vi "Render.vi"(8 "error in (no error)":errorcluster, 11 "XRay Axis Rails in":refnum<class "XRay Axis Rails.lvclass">) -> (0 "error out":errorcluster, 2 "Scene Object":refnum<vi>, 3 "XRay Axis Rails out":refnum<class "XRay Axis Rails.lvclass">)   [LabVIEW 2026, in "XRay Axis Rails.lvclass"]
uses:
  XRay Axis Rails.lvclass
  XRay Axis Rails.lvclass/XRay Axis Rails.ctl
  <vilib>/picture/picture.llb/imagedata.ctl
  <vilib>/picture/3D Picture Control/Object/Create Object (drawable).vi
  <vilib>/picture/3D Picture Control/Object/Add Object (reference).vi
  <vilib>/picture/3D Picture Control/Helpers/Apply Texture (reference).vi
  <vilib>/picture/3D Picture Control/NI_3D Picture Control.lvlib
panel:
  in  "Apply Mode":T1(ring)=enum."As a replacement"
  in  "error in (no error) 2":errorcluster
  in  "Translation 4":cluster{"X":sgl, "Y":sgl, "Z":sgl}={"X"=0.0, "Y"=9.0, "Z"=5.0}
  in  "Translation 3":cluster{"X":sgl, "Y":sgl, "Z":sgl}={"X"=0.0, "Y"=5.0, "Z"=5.0}
  in  "Translation 2":cluster{"X":sgl, "Y":sgl, "Z":sgl}={"X"=7.0, "Y"=7.5, "Z"=0.0}
  in  "Translation":cluster{"X":sgl, "Y":sgl, "Z":sgl}={"X"=4.0, "Y"=7.5, "Z"=0.0}
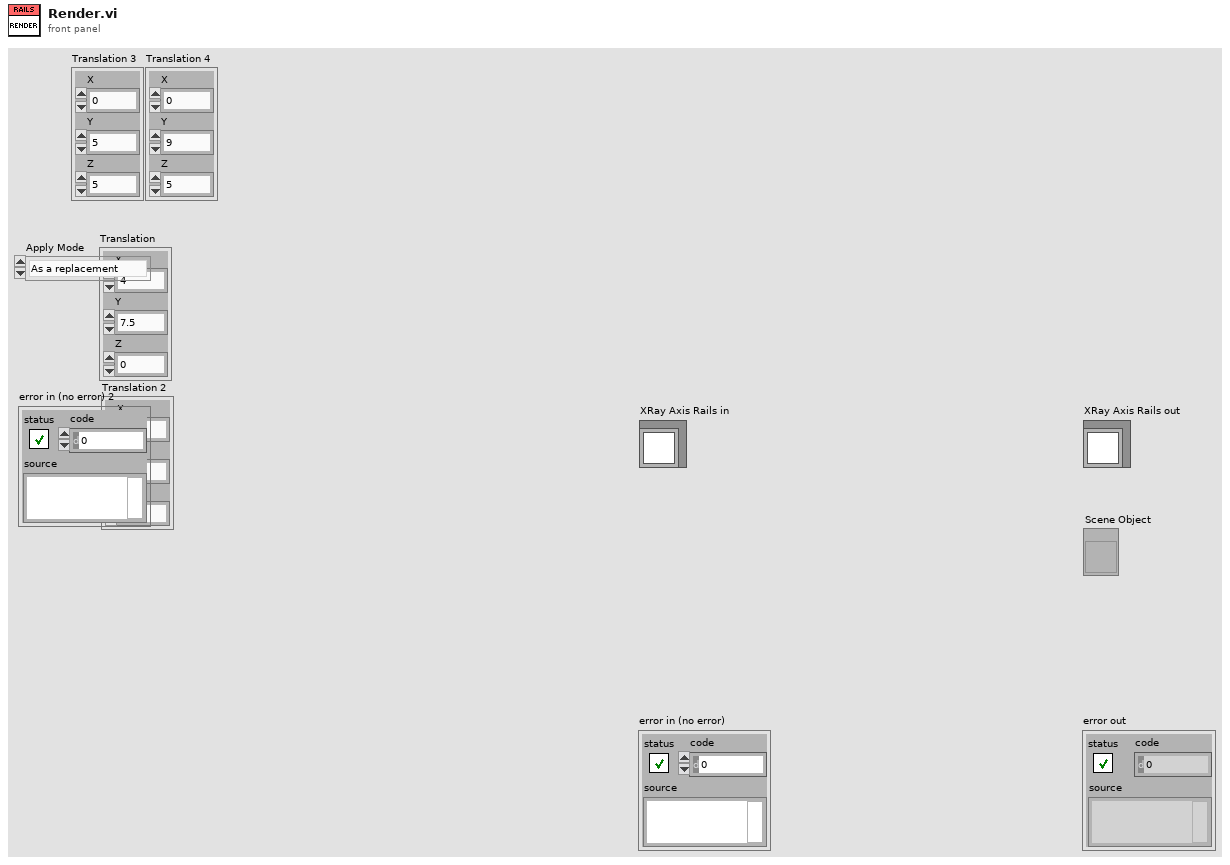
[diagram p1: front panel]
types:
  T1 = enum16{"As a Decal", "With Modulation", "With Blending", "As a replacement"}
  T2 = enum16{"No Filtration", "Linear Filtration", "Simple Mipmap Filtration", "Bilinear Filtration", "Trilinear Filtration"}
  T3 = enum16{"Inherit Value", "Points", "Wireframe", "Polygons"}
  T4 = typedef "imagedata.ctl" = cluster{"image type":i32, "image depth":i32, "image":u8[], "mask":u8[], "colors":u32[], "Rectangle":cluster{"left":i16, "top":i16, "right":i16, "bottom":i16}}
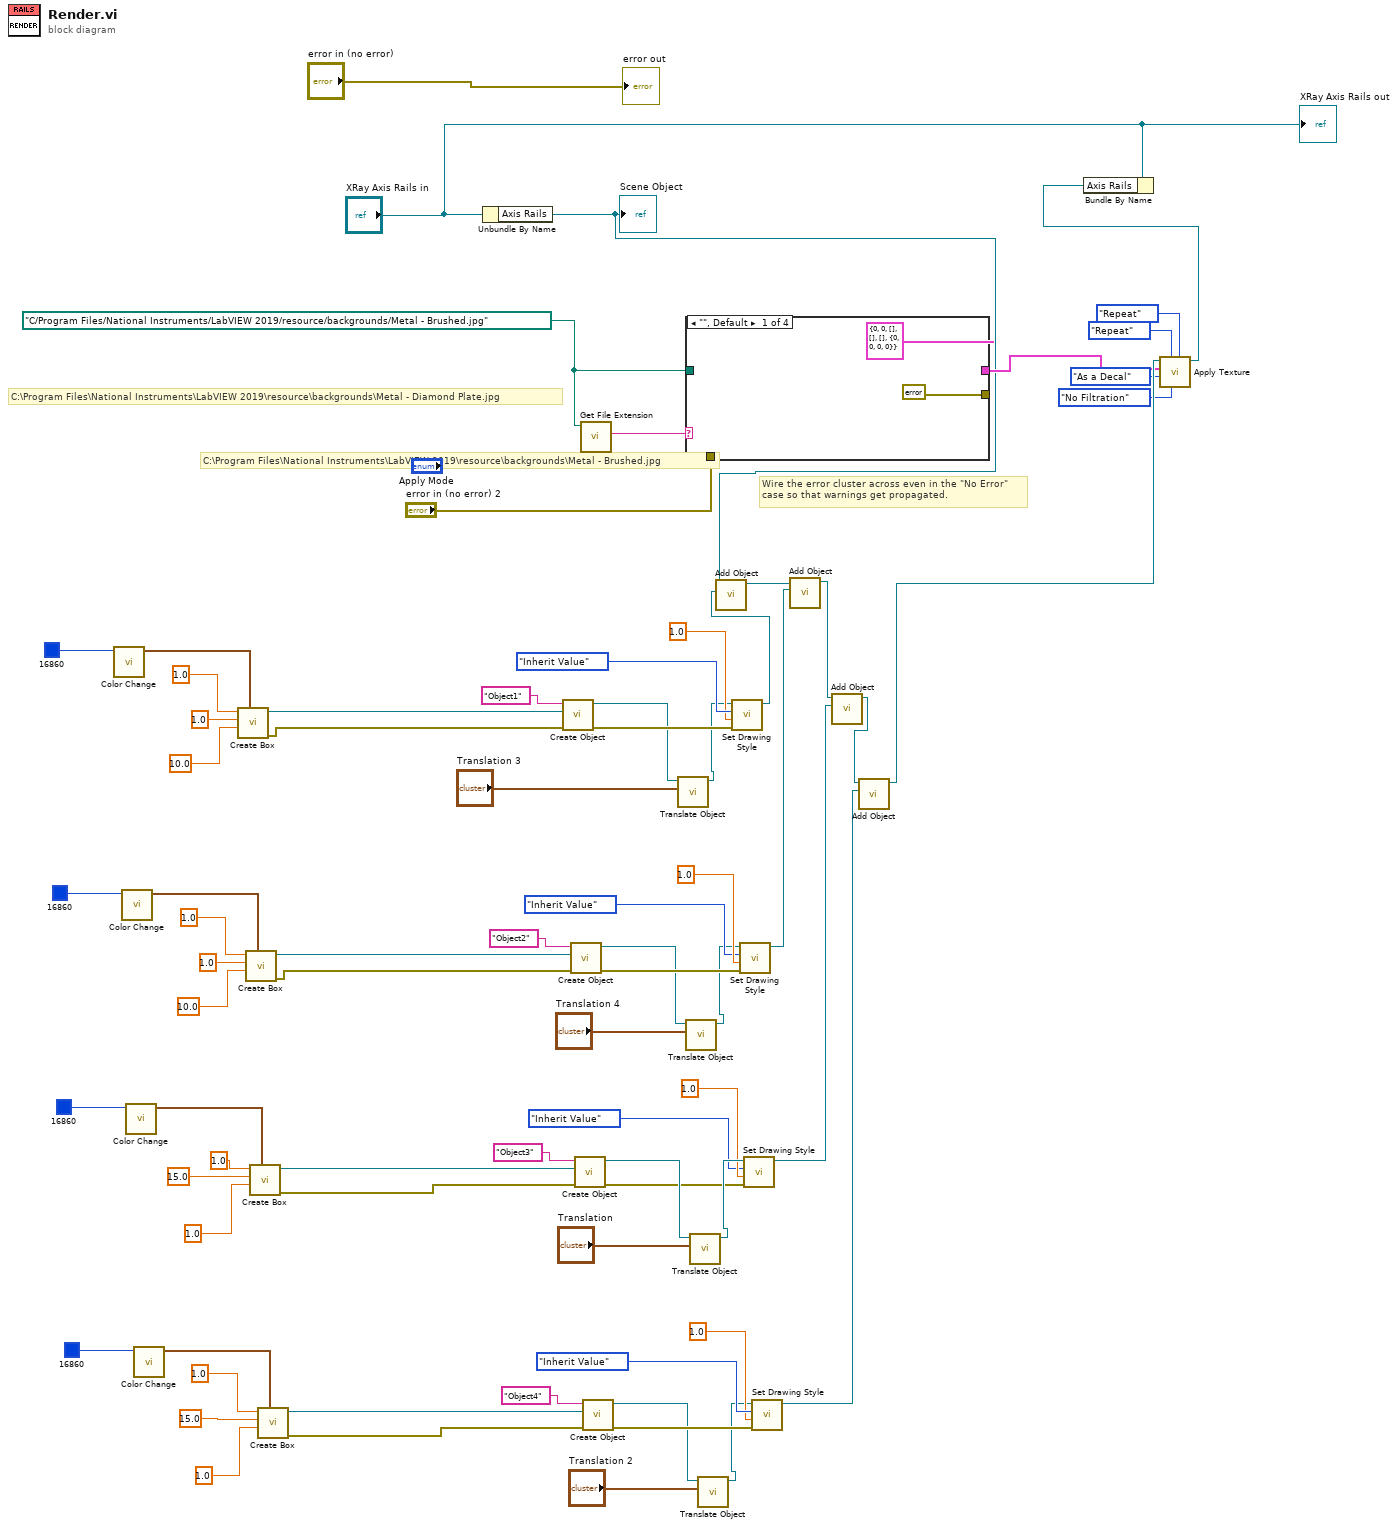
[diagram p0: block diagram]
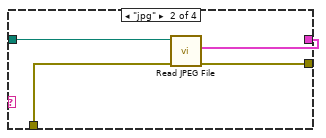
[diagram p2: hidden frame]
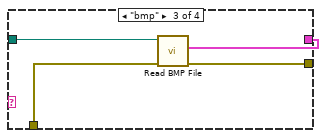
[diagram p3: hidden frame]
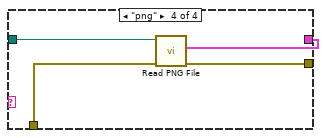
[diagram p4: hidden frame]
diagram:
  w11 = path "C:/Program Files/National Instruments/LabVIEW 2019/resource/backgrounds/Metal - Brushed.jpg" ("Path to Texture")
  # "C:\\Program Files\\National Instruments\\LabVIEW 2019\\resource\\backgrounds\\Metal - Brushed.jpg"
  # "C:\\Program Files\\National Instruments\\LabVIEW 2019\\resource\\backgrounds\\Metal - Diamond Plate.jpg"
  # "Wire the error cluster across even in the \"No Error\"\ncase so that warnings get propagated."
  n1 = call <vilib>:"Color Change.vi"("Color"=u32 16860) -> ("RGBA"=w74:cluster{"R":sgl, "G":sgl, "B":sgl, "A":sgl})  [unwired: 10 in]
  n2 = call <vilib>:"Color Change.vi"("Color"=u32 16860) -> ("RGBA"=w53:cluster{"R":sgl, "G":sgl, "B":sgl, "A":sgl})  [unwired: 10 in]
  n3 = call <vilib>:"Color Change.vi"("Color"=u32 16860) -> ("RGBA"=w23:cluster{"R":sgl, "G":sgl, "B":sgl, "A":sgl})  [unwired: 10 in]
  n4 = call <vilib>:"Color Change.vi"("Color"=u32 16860) -> ("RGBA"=w48:cluster{"R":sgl, "G":sgl, "B":sgl, "A":sgl})  [unwired: 10 in]
  n5 = call <vilib>:"Create Box.vi"("Color"=w74, "Length Z"=sgl 10.0 ("Box Length Z"), "Length Y"=sgl 1.0 ("Box Length Y"), "Length X"=sgl 1.0 ("Box Length X")) -> ("error out"=w72:errorcluster, "New Box Refnum"=w68:refnum<vi>)  [unwired: 6 in]
  n6 = call <vilib>:"Create Box.vi"("Color"=w53, "Length Z"=sgl 10.0 ("Box Length Z"), "Length Y"=sgl 1.0 ("Box Length Y"), "Length X"=sgl 1.0 ("Box Length X")) -> ("error out"=w55:errorcluster, "New Box Refnum"=w59:refnum<vi>)  [unwired: 6 in]
  n7 = call <vilib>:"Create Box.vi"("Color"=w23, "Length Z"=sgl 1.0 ("Box Length Z"), "Length Y"=sgl 15.0 ("Box Length Y"), "Length X"=sgl 1.0 ("Box Length X")) -> ("error out"=w25:errorcluster, "New Box Refnum"=w29:refnum<vi>)  [unwired: 6 in]
  n8 = call <vilib>:"Create Box.vi"("Color"=w48, "Length Z"=sgl 1.0 ("Box Length Z 3"), "Length Y"=sgl 15.0 ("Box Length Y 3"), "Length X"=sgl 1.0 ("Box Length X 3")) -> ("error out"=w46:errorcluster, "New Box Refnum"=w42:refnum<vi>)  [unwired: 6 in]
  n9 = Unbundle By Name("XRay Axis Rails in") -> ("Axis Rails"=w3:refnum<vi>)
  "Scene Object" <- w3
  n10 = call-poly <vilib>:"Create Object.vi"("error in (no error)"=w72, "Geometry"=w68, "Name"="Object1") -> ("error out"=w69:errorcluster, "Scene:New Object"=w50:refnum<vi>)  [unwired: 7 in]
  n11 = call-poly <vilib>:"Create Object.vi"("error in (no error)"=w55, "Geometry"=w59, "Name"="Object2") -> ("error out"=w58:errorcluster, "Scene:New Object"=w51:refnum<vi>)  [unwired: 7 in]
  n12 = call-poly <vilib>:"Create Object.vi"("error in (no error)"=w25, "Geometry"=w29, "Name"="Object3") -> ("error out"=w28:errorcluster, "Scene:New Object"=w30:refnum<vi>)  [unwired: 7 in]
  n13 = call <vilib>:"Get File Extension.vi"("file"=w11) -> ("lowercase file extension"=w10:string)  [unwired: 1 in, 9 out]
  n14 = call-poly <vilib>:"Create Object.vi"("error in (no error)"=w46, "Geometry"=w42, "Name"="Object4") -> ("error out"=w43:errorcluster, "Scene:New Object"=w41:refnum<vi>)  [unwired: 7 in]
  n15 = call <vilib>:"Translate Object.vi"("Translation"="Translation 3", "Scene.Object In"=w50) -> ("Scene.Object Out"=w16:refnum<vi>)  [unwired: 8 in, 1 out]
  n16 = case shown="\"\", Default" w10 {
    tunnel: [T4 {"image type"=0, "image depth"=0, "image"=[], "mask"=[], "colors"=[], "Rectangle"={"left"=0, "top"=0, "right"=0, "bottom"=0}} ("image data") w82 w86 w89] -> w8
    tunnel: [errorcluster {"status"=TRUE, "code"=5003, "source"="Invalid Picture file extension."} ("error out") w81 w85 w88] -> _
    tunnel: w11 -> [_ w80 w83 w90]
    tunnel: "error in (no error) 2" -> [_ w79 w84 w87]
    frame "", Default {
    }
    frame "jpg" {
      n17 = call <vilib>:"Read JPEG File.vi"("error in (no error)"=w79, "path to JPEG file"=w80) -> ("error out"=w81:errorcluster, "image data"=w82:T4)  [unwired: 8 out]
    }
    frame "bmp" {
      n18 = call <vilib>:"Read BMP File.vi"("error in (no error)"=w84, "path to BMP file"=w83) -> ("error out"=w85:errorcluster, "image data"=w86:T4)  [unwired: 8 out]
    }
    frame "png" {
      n19 = call <vilib>:"Read PNG File.vi"("error in (no error)"=w87, "path to PNG file"=w90) -> ("error out"=w88:errorcluster, "image data"=w89:T4)  [unwired: 8 out]
    }
  }
  n20 = call <vilib>:"Translate Object.vi"("Translation"="Translation 4", "Scene.Object In"=w51) -> ("Scene.Object Out"=w15:refnum<vi>)  [unwired: 8 in, 1 out]
  n21 = call <vilib>:"Translate Object.vi"("Translation"="Translation", "Scene.Object In"=w30) -> ("Scene.Object Out"=w31:refnum<vi>)  [unwired: 8 in, 1 out]
  n22 = call <vilib>:"Translate Object.vi"("Translation"="Translation 2", "Scene.Object In"=w41) -> ("Scene.Object Out"=w40:refnum<vi>)  [unwired: 8 in, 1 out]
  n23 = call <vilib>:"Set Drawing Style.vi"("error in (no error)"=w69, "Size"=1.0, "Mode"=T3."Inherit Value" ("Draw Mode"), "Scene Object In"=w16) -> ("Scene Object Out"=w14:refnum<vi>)  [unwired: 6 in, 1 out]
  n24 = call-poly <vilib>:"Add Object.vi"("New Object In"=w14, "Scene Object In"=w3) -> ("Scene Object Out"=w13:refnum<vi>)  [unwired: 7 in, 2 out]
  n25 = call <vilib>:"Set Drawing Style.vi"("error in (no error)"=w58, "Size"=1.0, "Mode"=T3."Inherit Value" ("Draw Mode"), "Scene Object In"=w15) -> ("Scene Object Out"=w21:refnum<vi>)  [unwired: 6 in, 1 out]
  n26 = call <vilib>:"Set Drawing Style.vi"("error in (no error)"=w28, "Size"=1.0, "Mode"=T3."Inherit Value" ("Draw Mode"), "Scene Object In"=w31) -> ("Scene Object Out"=w19:refnum<vi>)  [unwired: 6 in, 1 out]
  n27 = call <vilib>:"Set Drawing Style.vi"("error in (no error)"=w43, "Size"=1.0, "Mode"=T3."Inherit Value" ("Draw Mode"), "Scene Object In"=w40) -> ("Scene Object Out"=w17:refnum<vi>)  [unwired: 6 in, 1 out]
  n28 = call-poly <vilib>:"Add Object.vi"("New Object In"=w21, "Scene Object In"=w13) -> ("Scene Object Out"=w20:refnum<vi>)  [unwired: 7 in, 2 out]
  n29 = call-poly <vilib>:"Add Object.vi"("New Object In"=w19, "Scene Object In"=w20) -> ("Scene Object Out"=w18:refnum<vi>)  [unwired: 7 in, 2 out]
  n30 = call-poly <vilib>:"Add Object.vi"("New Object In"=w17, "Scene Object In"=w18) -> ("Scene Object Out"=w9:refnum<vi>)  [unwired: 7 in, 2 out]
  n31 = call-poly <vilib>:"Apply Texture.vi"("Vertical Wrap Mode"=enum16{"Clamp", "Repeat"}."Repeat", "Filter Mode"=T2."No Filtration", "Horizontal Wrap Mode"=enum16{"Clamp", "Repeat"}."Repeat", "Apply Mode"=T1."As a Decal", "Image Data"=w8, "Scene Object In"=w9) -> ("Scene Object Out"=w1:refnum<vi>)  [unwired: 3 in, 2 out]
  n32 = Bundle By Name(cluster="XRay Axis Rails in", "Axis Rails"=w1) -> ()  [unwired: 1 out]
  "error out" <- "error in (no error)"
  "XRay Axis Rails out" <- "XRay Axis Rails in"
